vi "normalize_array_advanced.vi"(10 "i32_ar_first_and_last_pixel":i32[](array[numeric]), 11 "unwrapped array":i16[](array[numeric])) -> (3 "normalized unwrapped array":u8[](array[numeric]))   [LabVIEW 2011]
doc: "Normalizes the row to values between 0 and 255 as well as set the mask values to zero."
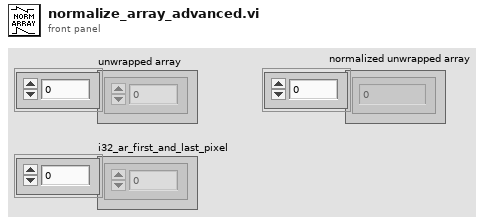
[diagram p1: front panel]
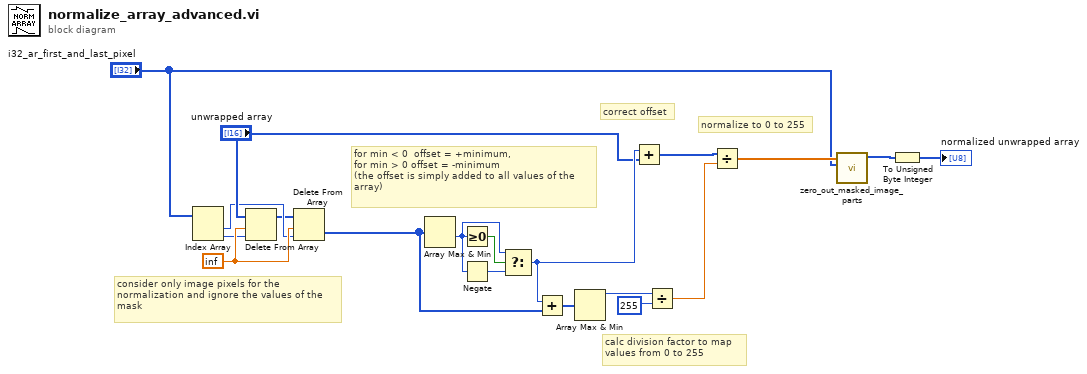
[diagram p0: block diagram]
diagram:
  w8 = inf
  # "normalize to 0 to 255"
  # "calc division factor to map\nvalues from 0 to 255"
  # "consider only image pixels for the \nnormalization and ignore the values of the\nmask"
  # "for min < 0  offset = +minimum,\nfor min > 0 offset = -minimum\n(the offset is simply added to all values of the \narray)"
  # "correct offset"
  n1 = Index Array(array="i32_ar_first_and_last_pixel") -> (element #1=w7:i32, element #2=w5:i32)  [unwired: 2 in]
  n2 = Delete From Array(array="unwrapped array", length=w8, index=w5) -> (array with subset deleted=w6:i16[])  [unwired: 1 out]
  n3 = Delete From Array(array=w6, length=w8, index=w7) -> (deleted portion=w12:i16[])  [unwired: 1 out]
  n4 = Array Max & Min(array=w12) -> (min value=w11:i16)  [unwired: 3 out]
  n5 = Greater Or Equal To 0?(x=w11) -> (x >= 0?=w9:bool)
  n6 = Negate(x=w11) -> (-x=w10:i16)
  n7 = Select(t=w11, s=w9, f=w10) -> (s? t:f=w17:i16)
  n8 = Add(x=w17, y=w12) -> (x+y=w15:i16[])
  n9 = Array Max & Min(array=w15) -> (max value=w14:i16)  [unwired: 3 out]
  n10 = Add(x=w17, y="unwrapped array") -> (x+y=w18:i16[])
  n11 = Divide(x=w14, y=i16 255) -> (x/y=w19:dbl)
  n12 = Divide(x=w18, y=w19) -> (x/y=w4:dbl[])
  n13 = call "zero_out_masked_image_parts.vi"("i32_ar_first_and_last_pixel"="i32_ar_first_and_last_pixel", "unwrapped_Array"=w4) -> ("Array out"=w2:i16[])  [unwired: 9 in]
  n14 = To Unsigned Byte Integer(number=w2) -> (unsigned 8bit integer=→"normalized unwrapped array":u8[])
